vi "ProdaNG.Example.AddProductComponent.vi"() -> ()   [LabVIEW 2016]
uses:
  Controls/ProdaNG.ProcessResult.ctl
  Controls/ProdaNG.ProcessStepResult.ctl
  Controls/ProdaNG.Product.ctl
  Controls/ProdaNG.Identification.ctl
panel:
  out "Identification 2":T1
  out "Identification":T1
  in  "systemName 2":string="M110"
  in  "wabcoNumber 2":string="4154064040"
  out "Product out 2":T2
  out "Product out 1":T2
  out "Status 2":T3
  out "Status 1":T3
  in  "serialNumber 2":string="1510130001"
  out "source":string
  in  "serialNumber 1":string="30010025161214"
  in  "systemName 1":string="M80"
  out "ErrCode":i32
  out "error out":errorcluster
  in  "error in (no error)":errorcluster
  in  "wabcoNumber 1":string="4430203001"
  out "DataBase time":string
  in  "Connection string":string="lcptb/lcptb@PRODA_WPK"
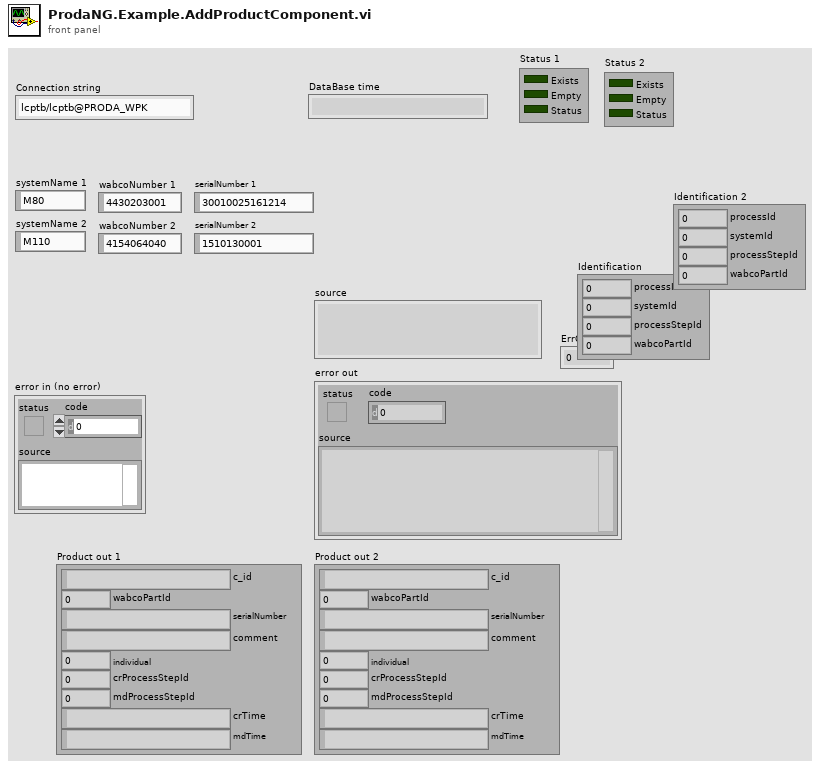
[diagram p1: front panel]
types:
  T1 = typedef "ProdaNG.Identification.ctl" = cluster{"processId":i32, "systemId":i32, "processStepId":i32, "wabcoPartId":i32}
  T2 = typedef "ProdaNG.Product.ctl" = cluster{"c_id":string, "wabcoPartId":i32, "serialNumber":string, "comment":string, "individual":i32, "crProcessStepId":i32, "mdProcessStepId":i32, "crTime":string, "mdTime":string}
  T3 = cluster{"Exists":bool, "Empty":bool, "Status":bool}
  T4 = typedef "ProdaNG.ProcessStepResult.ctl" = cluster{"c_id":string, "processResultId":string, "processStepId":i32, "statusId":i32, "operatorId":i32, "startTime":string, "endTime":string}
  T5 = typedef "ProdaNG.ProcessResult.ctl" = cluster{"c_id":string, "productId":string, "processId":i32, "statusId":i32, "startTime":string, "endTime":string}
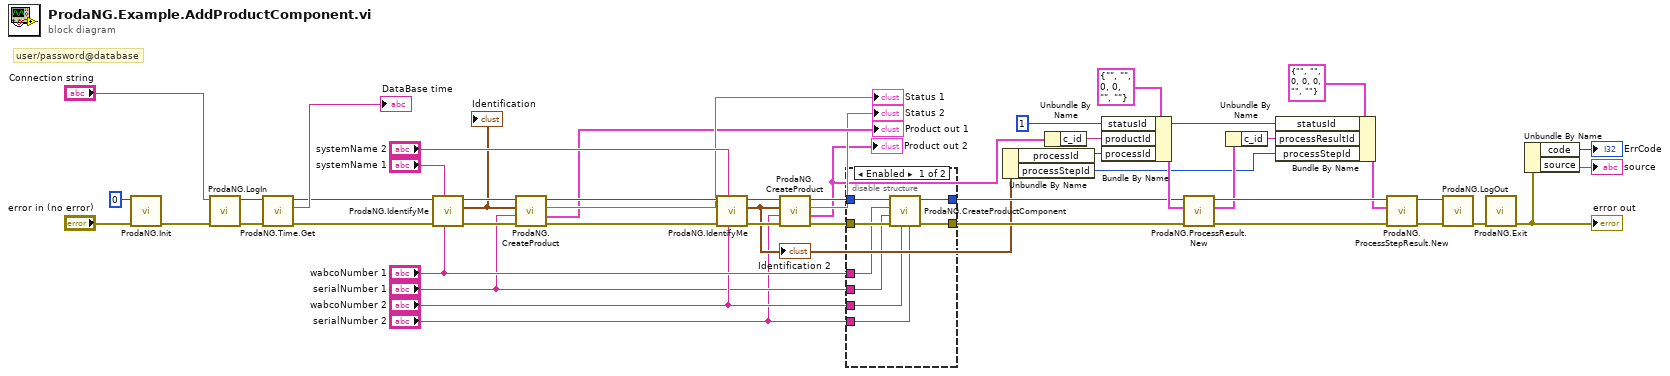
[diagram p0: block diagram]
diagram:
  w1 = 1 ("Step.statusId")
  # "user/password@database"
  n1 = call "ProdaNG.Init.vi"("error in (no error)"="error in (no error)", "numContexts (0: unlimited)"=0 ("numContexts")) -> ("error out"=w48:errorcluster)  [unwired: 9 in]
  n2 = call "ProdaNG.LogIn.vi"("error in"=w48, "ConnectionString"="Connection string") -> ("error out"=w44:errorcluster, "dbHandle"=w45:i32)  [unwired: 7 in, 1 out]
  n3 = call "ProdaNG.Time.Get.vi"("error in"=w44, "dbHandleIn"=w45) -> ("error out"=w39:errorcluster, "timeStr"=→"DataBase time":string, "dbHandle"=w40:i32)  [unwired: 5 in, 1 out]
  n4 = call "ProdaNG.IdentifyMe.vi"("wabcoNumber"="wabcoNumber 1", "systemName"="systemName 1", "error in"=w39, "dbHandleIn"=w40) -> ("error out"=w36:errorcluster, "Identification"=w9:T1, "dbHandle"=w37:i32)  [unwired: 5 in]
  "Identification" <- w9
  n5 = call "ProdaNG.CreateProduct.vi"("error in (no error)"=w36, "serialNumber"="serialNumber 1", "ID"=w9, "dbHandle"=w37) -> ("error out"=w30:errorcluster, "Product out"=→"Product out 1":T2, 2:→"Status 1", "dbHandle out"=w31:i32)  [unwired: 4 in]
  n6 = call "ProdaNG.IdentifyMe.vi"("wabcoNumber"="wabcoNumber 2", "systemName"="systemName 2", "error in"=w30, "dbHandleIn"=w31) -> ("error out"=w28:errorcluster, "Identification"=w5:T1, "dbHandle"=w29:i32)  [unwired: 5 in]
  "Identification 2" <- w5
  n7 = call "ProdaNG.CreateProduct.vi"("error in (no error)"=w28, "serialNumber"="serialNumber 2", "ID"=w5, "dbHandle"=w29) -> ("error out"=w34:errorcluster, "Product out"=w2:T2, 2:→"Status 2", "dbHandle out"=w33:i32)  [unwired: 4 in]
  "Product out 2" <- w2
  n8 = disable-structure shown="Enabled" {
    disable-tunnel: w34 -> [w57 w59]
    disable-tunnel: w33 -> [w56 w58]
    disable-tunnel: [w55 w58] -> w19
    disable-tunnel: [w54 w59] -> w18
    disable-tunnel: "wabcoNumber 1" -> [w53 _]
    disable-tunnel: "serialNumber 1" -> [w52 _]
    disable-tunnel: "wabcoNumber 2" -> [w51 _]
    disable-tunnel: "serialNumber 2" -> [w50 _]
    frame Enabled {
      n9 = call "ProdaNG.CreateProductComponent.vi"("component serialNo"=w50, "component wabcoNo"=w51, "error in (no error)"=w57, "product serialNo"=w52, "product wabcoNo"=w53, "dbHandle"=w56) -> ("error out"=w54:errorcluster, "dbHandle out"=w55:i32)  [unwired: 4 in]
    }
    frame Disabled {
    }
  }
  n10 = Unbundle By Name(w5) -> ("processId"=w11:i32, "processStepId"=w10:i32)
  n11 = Unbundle By Name(w2) -> ("c_id"=w24:string)
  n12 = Bundle By Name(cluster=T5 {"c_id"="", "productId"="", "processId"=0, "statusId"=0, "startTime"="", "endTime"=""} ("ProcessResult"), "statusId"=w1, "productId"=w24, "processId"=w11) -> (w22:T5)
  n13 = call "ProdaNG.ProcessResult.New.vi"("error in (no error)"=w18, "ProcessResult"=w22, "dbHandle"=w19) -> ("error out"=w26:errorcluster, "ProcessResult out"=w20:T5, "dbHandle"=w25:i32)  [unwired: 6 in]
  n14 = Unbundle By Name(w20) -> ("c_id"=w23:string)
  n15 = Bundle By Name(cluster=T4 {"c_id"="", "processResultId"="", "processStepId"=0, "statusId"=0, "operatorId"=0, "startTime"="", "endTime"=""} ("ProcessStepResult"), "statusId"=w1, "processResultId"=w23, "processStepId"=w10) -> (w21:T4)
  n16 = call "ProdaNG.ProcessStepResult.New.vi"("error in (no error)"=w26, "ProcessStepResult"=w21, "dbHandle"=w25) -> ("error out"=w17:errorcluster, "dbHandle"=w16:i32)  [unwired: 6 in, 1 out]
  n17 = call "ProdaNG.LogOut.vi"("error in"=w17, "dbHandleIn"=w16) -> ("error out"=w49:errorcluster)  [unwired: 9 in]
  n18 = call "ProdaNG.Exit.vi"("error in (no error)"=w49) -> ("error out"=w32:errorcluster)  [unwired: 10 in]
  "error out" <- w32
  n19 = Unbundle By Name(w32) -> ("code"=→"ErrCode":i32, "source"=→"source":string)
